vi "Limit Theta Range.vi"(1 "States In":T1 format="%.4f") -> (0 "States Out":T1 format="%.4f")   [LabVIEW 2018]
uses:
  States.ctl
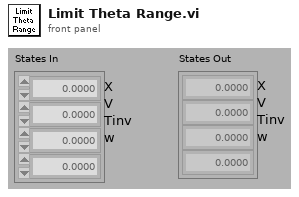
[diagram p1: front panel]
types:
  T1 = typedef "States.ctl" = dbl[]
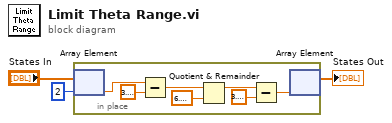
[diagram p0: block diagram]
diagram:
  n1 = in-place {
    n2 = in-place-array #1("States In", 2) -> (w4:dbl)
    n3 = Subtract(x=w4, y=3.141592653589793) -> (x-y=w6:dbl)
    n4 = Quotient & Remainder(x=w6, y=6.283185307179586) -> (x-y*floor(x/y)=w7:dbl)  [unwired: 1 out]
    n5 = Subtract(x=w7, y=3.141592653589793) -> (x-y=w5:dbl)
    n6 = in-place-array #1(w5) -> (→"States Out":T1)  [unwired: 1 out]
  }
